vi "parseStatus.vi"(8 "error in (no error)":errorcluster, 9 "timeout":bool=TRUE, 10 "Message":string, 11 "tcpDevice in":refnum<class "tcpDevice.lvclass">) -> (0 "error out":errorcluster, 2 "status":T1, 3 "tcpDevice out":refnum<class "tcpDevice.lvclass">)   [LabVIEW 2016, in "tcpDevice.lvclass"]
uses:
  tcpDevice.lvclass
  typedefs/deviceStatus.ctl
  typedefs/statusEnum.ctl
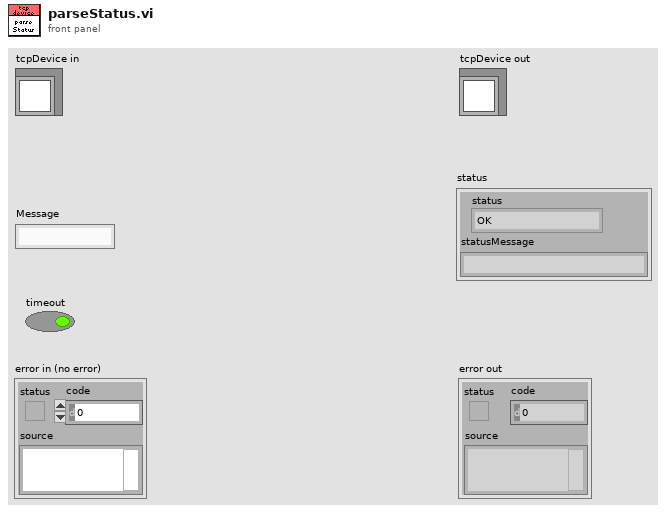
[diagram p1: front panel]
types:
  T1 = typedef "deviceStatus.ctl" = cluster{"status":T2, "statusMessage":string}
  T2 = typedef "statusEnum.ctl" = enum16{"OK", "TIMEOUT", "MSGERROR"}
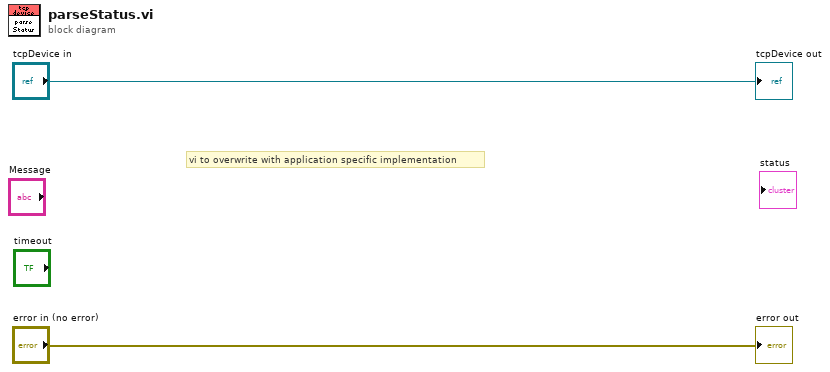
[diagram p0: block diagram]
diagram:
  # "vi to overwrite with application specific implementation"
  "error out" <- "error in (no error)"
  "tcpDevice out" <- "tcpDevice in"
